vi "AAnT.vi"(0 "Archivo de\nreferencias (.csv)":path, 4 "FEATS":path, 5 "ARCHIVO\nTDMS":path, 7 "Largo de ventada temporal en N samples":dbl=4410.0, 9 "Canal":string[](array[string])=["Sound Pressure_0"], 11 "frequency range":T1={"low band"=enum."20 Hz", "high band"=enum."20000 Hz"}) -> ()   [LabVIEW 2017]
uses:
  <vilib>/Waveform/WDTOps.llb/WDT Get Waveform Subset DBL.vi
  <vilib>/addons/Sound and Vibration/svt_Octave_2014 standard/SVT Fractional-octave Analysis (1 Ch).vi
  <vilib>/addons/Sound and Vibration/svt_Level/SVT Sound Level (1 Ch).vi
  <vilib>/Utility/file.llb/Write Delimited Spreadsheet (string).vi
  <vilib>/addons/Sound and Vibration/svt_Level/SoundVib_SoundLevel.lvlib
  <vilib>/addons/Sound and Vibration/svt_Octave/SoundVib_Octave_2014 standard.lvlib
panel:
  out "F-format string":string[][](array[string])
  out "Array":dbl[][](array[numeric])
  out "Para el CSV, excepto fecha y hora":string[][](array[string])
  out "TO CSV.":string[][](array[string])
  out "ETIQUETAS":string[](array[string])
  out "BANDAS":dbl[][](array[numeric])
  out "Dynamic Data Type":dbl
  out "Samples \npor Objeto":waveform(dbl)
  out "Multiplot \noctave graph":T2(graph)
  out "Secciones":waveform(dbl)[](array[waveform])
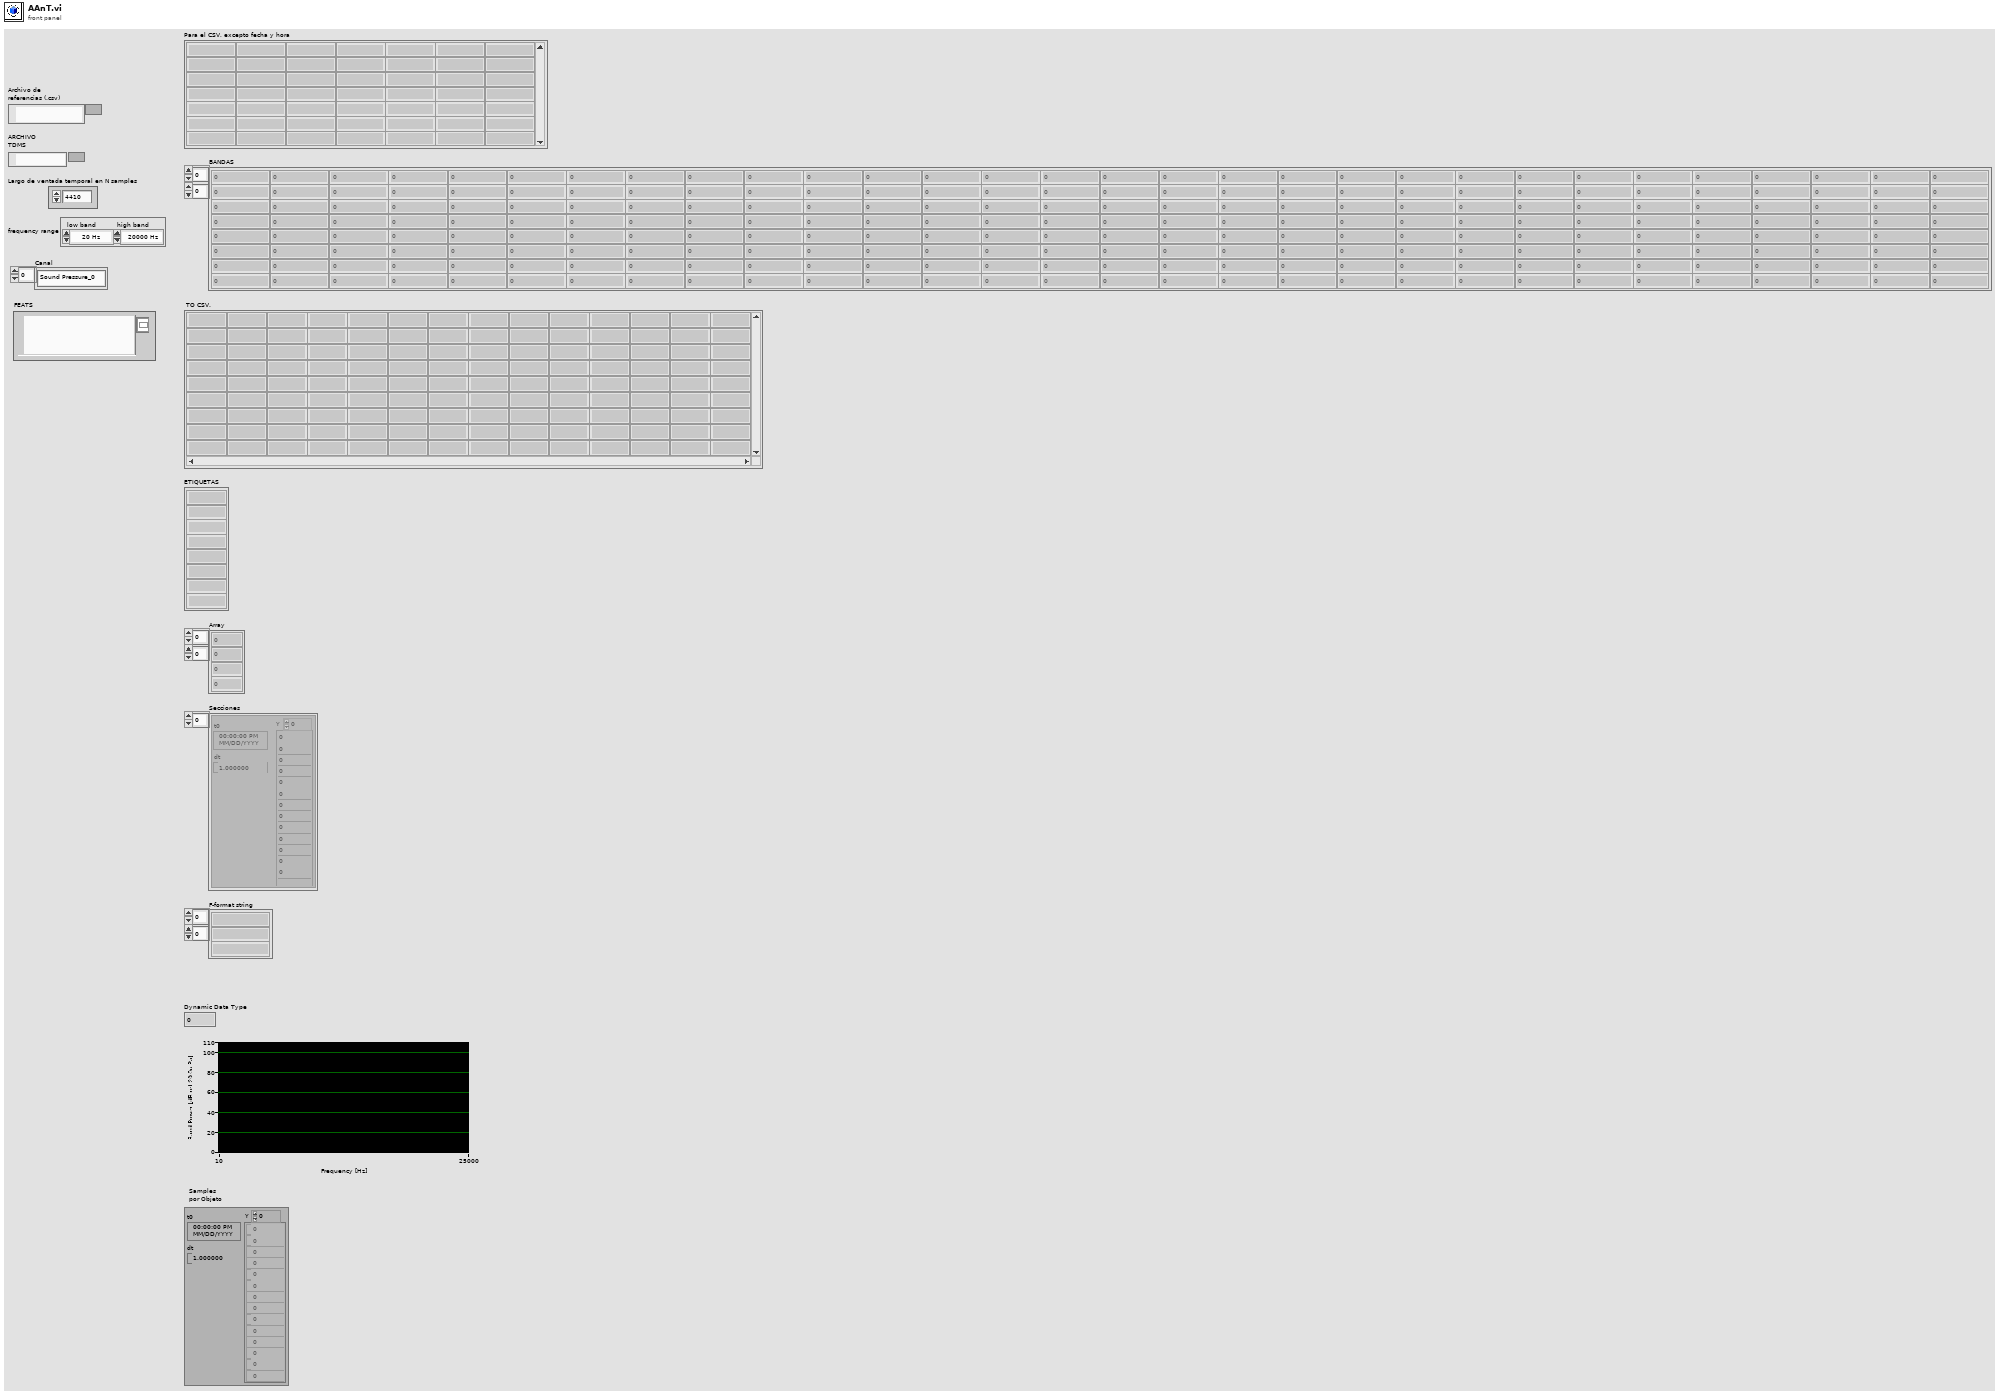
[diagram p1: front panel]
types:
  T1 = cluster{"low band":enum16{"20 Hz", "25 Hz", "31.5 Hz", "40 Hz", "50 Hz", "63 Hz", "80 Hz", "100 Hz", "125 Hz", "160 Hz", "200 Hz", "250 Hz", "315 Hz", "400 Hz", "500 Hz", "630 Hz", "800 Hz", "1000 Hz", "1250 Hz", "1600 Hz", "2000 Hz", "2500 Hz", "3150 Hz", "4000 Hz", "5000 Hz", "6300 Hz", "8000 Hz", "10000 Hz", "12500 Hz", "16000 Hz", "20000 Hz"}, "high band":enum16{"20 Hz", "25 Hz", "31.5 Hz", "40 Hz", "50 Hz", "63 Hz", "80 Hz", "100 Hz", "125 Hz", "160 Hz", "200 Hz", "250 Hz", "315 Hz", "400 Hz", "500 Hz", "630 Hz", "800 Hz", "1000 Hz", "1250 Hz", "1600 Hz", "2000 Hz", "2500 Hz", "3150 Hz", "4000 Hz", "5000 Hz", "6300 Hz", "8000 Hz", "10000 Hz", "12500 Hz", "16000 Hz", "20000 Hz"}}
  T2 = cluster{"nominal frequencies [Hz]":dbl[], "band power":dbl[]}
  T3 = enum16{"open", "open or create", "create or replace", "create", "open (read-only)"}
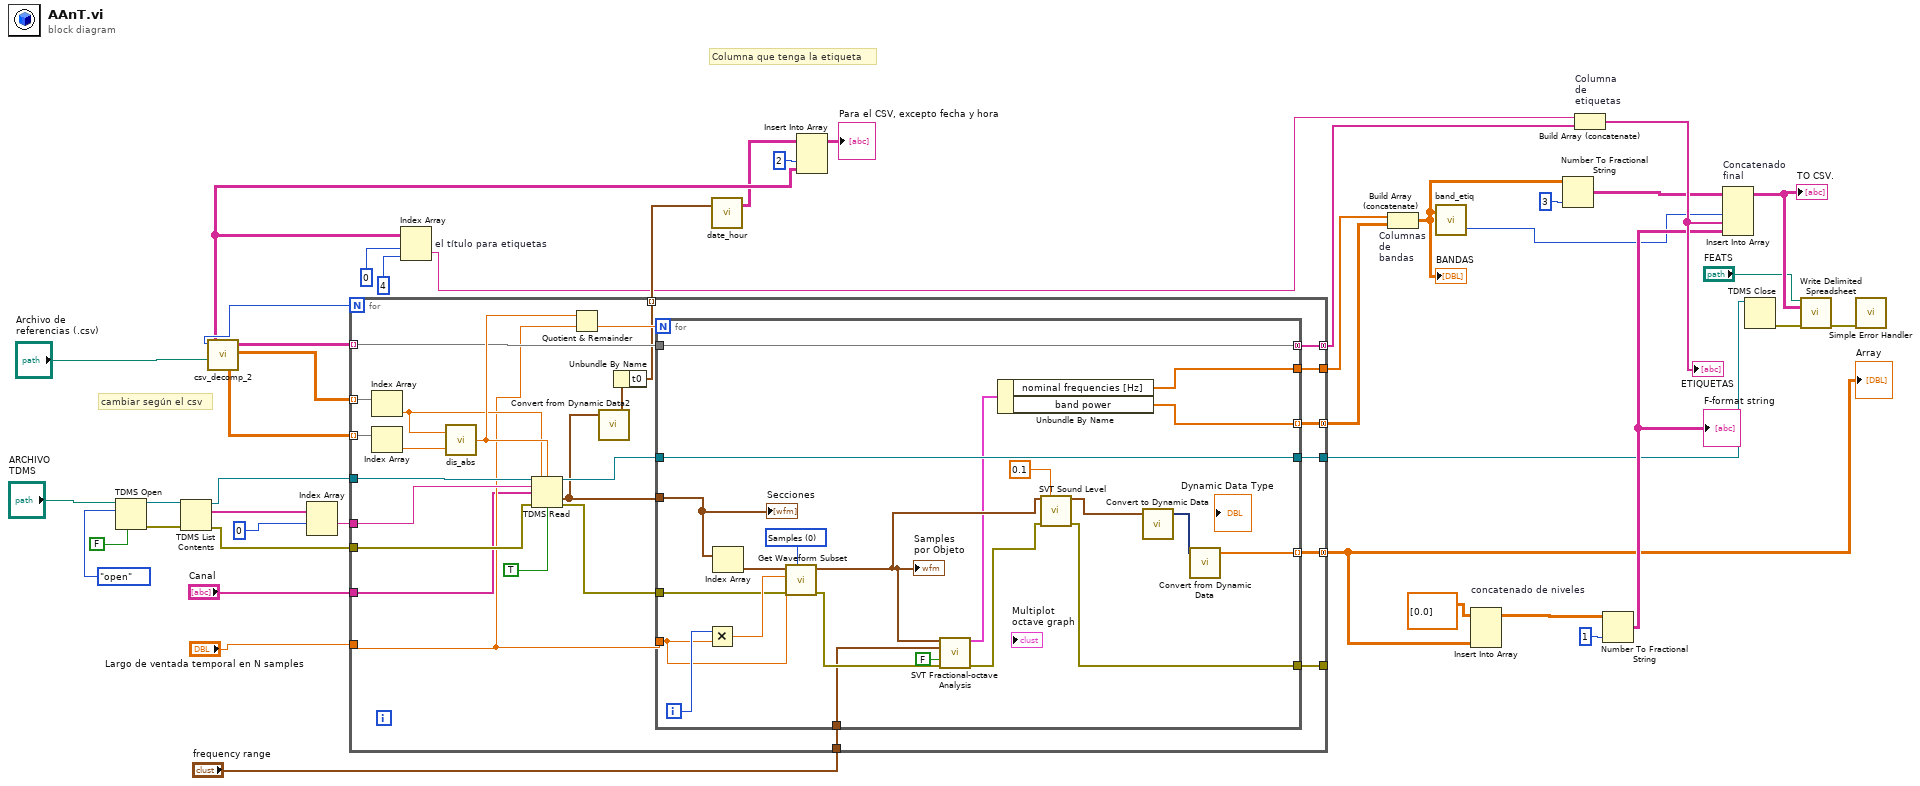
[diagram p0: block diagram]
diagram:
  # "cambiar según el csv"
  # "Columna que tenga la etiqueta"
  n1 = TDMS Open(6:FALSE ("disable buffering? (T)"), 10:T3."open" ("operation (0:open)"), 11:"ARCHIVO\nTDMS") -> (0:w6:errorcluster, 3:w29:refnum<k34>)  [unwired: 4 in]
  n2 = TDMS List Contents(4:w6, 7:w29) -> (0:w31:errorcluster, 2:w30:string[], 3:w7:refnum<k34>)  [unwired: 1 in, 1 out]
  n3 = call "csv_decomp_2.vi"("Archivo de referencias (.csv)"="Archivo de\nreferencias (.csv)") -> ("finales"=w36:dbl[][], "iniciales"=w37:dbl[][], "etiquetas"=w35:string[][], "# dimención"=w34:i32, "Lectura CSV"=w32:string[][])  [unwired: 2 in]
  n4 = Index Array(array=w30, index #1=0 ("index")) -> (element #1=w9:string)  [unwired: 1 in, 1 out]
  n5 = for {
    N: w34 -> [_]
    tunnel: w37 -> [w66] mode=indexing
    tunnel: w36 -> [w67] mode=indexing
    tunnel: w35 -> [w55] mode=indexing
    tunnel: w7 -> [w68]
    tunnel: w31 -> [w61]
    tunnel: w9 -> [w69]
    tunnel: [w59] -> w10
    tunnel: [w58] -> w11
    tunnel: [w57] -> w12 mode=concatenating
    tunnel: [w56] -> _
    tunnel: [w54] -> w16 mode=concatenating
    tunnel: "Largo de ventada temporal en N samples" -> [w51]
    tunnel: [w48] -> w25 mode=indexing
    tunnel: [w47] -> w39 mode=concatenating
    tunnel: "Canal" -> [w46]
    tunnel: "frequency range" -> [w45]
    n6 = Index Array(array=w66) -> (element=w53:dbl)  [unwired: 1 in]
    n7 = Index Array(array=w67) -> (element=w52:dbl)  [unwired: 1 in]
    n8 = call "dis_abs.vi"("Numeric in"=w52, "Numeric 3"=w53) -> ("distancia abs entre dos números"=w62:dbl)
    n9 = TDMS Read(0:w68, 1:w53, 2:w62, 5:w69, 7:w46, 11:w61, 13:TRUE ("return channels in file order? (F)")) -> (4:w65:refnum<k34>, 10:w50:waveform(dbl)[], 15:w60:errorcluster)  [unwired: 1 in, 3 out]
    n10 = Quotient & Remainder(x=w62, y=w51) -> (floor(x/y)=w63:dbl)  [unwired: 1 out]
    n11 = call "Convert from Dynamic Data2"("Dynamic Data Type"=w50) -> ("Waveform"=w49:waveform(dbl))  [unwired: 3 in]
    n12 = Unbundle By Name(w49) -> ("t0"=w48:timestamp)
    n13 = for {
      N: w63 -> [_]
      tunnel: w65 -> [w86]
      tunnel: w50 -> [w80]
      tunnel: w60 -> [w87]
      tunnel: [w77] -> w56
      tunnel: [w86] -> w59
      tunnel: [w85] -> w58
      tunnel: [w84] -> w57 mode=indexing
      tunnel: w55 -> [w83]
      tunnel: [w83] -> w54 mode=concatenating
      tunnel: w51 -> [w81]
      tunnel: [w72] -> w47 mode=indexing
      tunnel: w45 -> [w70]
      i -> [w82]
      w89 = u16 0 items=["Samples", "Relative Time"] ("start/duration format")
      n14 = Multiply(x=w82, y=w81) -> (x*y=w88:dbl)
      n15 = Index Array(array=w80) -> (element=w90:waveform(dbl))  [unwired: 1 in]
      n16 = call-poly <vilib>:"Get Waveform Subset.vi"("start/duration format"=w89, "error in (no error)"=w87, "duration"=w81, "start samples/time"=w88, "waveform in"=w90) -> ("error out"=w91:errorcluster, "waveform out"=w79:waveform(dbl))  [unwired: 1 in, 2 out]
      "Samples \npor Objeto" <- w79
      n17 = call-poly <vilib>:"SVT Fractional-octave Analysis.vi"("scaled signal [EU]"=w79, "frequency range [Hz]"=w70, "dB On (T)"=FALSE, "error in (no error)"=w91) -> ("octave spectrum"=w75:T2, "error out"=w78:errorcluster)  [unwired: 6 in, 4 out]
      n18 = Unbundle By Name(w75) -> ("nominal frequencies [Hz]"=w85:dbl[], "band power"=w84:dbl[])
      n19 = call-poly <vilib>:"SVT Sound Level.vi"("scaled signal [EU]"=w79, "integration time [s]"=0.1, "error in (no error)"=w78) -> ("Leq sound level [dB EU]"=w74:waveform(dbl), "error out"=w77:errorcluster)  [unwired: 7 in, 4 out]
      n20 = call "Convert to Dynamic Data"("Array"=w74) -> ("Dynamic Data Type"=w73:dynamicdata)  [unwired: 3 in]
      n21 = call "Convert from Dynamic Data"("Dynamic Data Type"=w73) -> ("Array"=w72:dbl[])  [unwired: 3 in]
      "Secciones" <- w80
    }
  }
  "Array" <- w39
  n22 = Index Array "el título para etiquetas"(array=w32, index (row)=0 ("disabled index (row)"), index (col)=4 ("disabled index (col)")) -> (element=w19:string)
  n23 = call "date_hour.vi"("Array"=w25) -> ("appended array"=w26:string[][])  [unwired: 1 in, 1 out]
  n24 = Insert Into Array(array=w26, index (col)=2 ("disabled index (col)"), new element=w32) -> (→"Para el CSV, excepto fecha y hora":string[][])  [unwired: 1 in]
  n25 = Build Array (concatenate) "Columnas \nde\nbandas"(w11, w12) -> (w22:dbl[][])
  "BANDAS" <- w22
  n26 = call "band_etiq.vi"("Array de entrada"=w22) -> ("Numeric"=w23:i32)  [unwired: 1 in, 1 out]
  n27 = Insert Into Array "concatenado de niveles"(array=dbl[][] [[0.0]], new element=w39) -> (w40:dbl[][])  [unwired: 2 in]
  n28 = Number To Fractional String(number=w22, precision (6)=i16 3) -> (F-format string=w21:string[][])  [unwired: 2 in]
  n29 = Build Array (concatenate) "Columna \nde \netiquetas"(w19, w16) -> (w44:string[])
  "ETIQUETAS" <- w44
  n30 = Number To Fractional String(number=w40, precision (6)=i16 1) -> (F-format string=w42:string[][])  [unwired: 2 in]
  "F-format string" <- w42
  n31 = Insert Into Array "Concatenado \nfinal"(array=w21, index (col)=w23, new element #1=w44, new element #2=w42) -> (w43:string[][])  [unwired: 1 in]
  "TO CSV." <- w43
  n32 = TDMS Close(11:w10) -> (0:w14:errorcluster)  [unwired: 1 in, 1 out]
  n33 = call-poly <vilib>:"Write Delimited Spreadsheet.vi"("file path (dialog if empty)"="FEATS", "2D data"=w43, "error in (no error)"=w14) -> ("error out"=w15:errorcluster)  [unwired: 11 in, 1 out]
  n34 = call <vilib>:"Simple Error Handler.vi"("error in (no error)"=w15) -> ()  [unwired: 4 in, 5 out]
